vi "Memory Benchmark.vi"(5 "Show Cache Lines (F)":bool, 7 "Show Peak Bandwidth (F)":bool, 9 "Transfers (500)":i32=500, 10 "End Size":u64=50000000 format="%.0pB", 11 "Start Size":u64=1000 format="%.0pB") -> (3 "Memory Bandwidth":cluster{"X":dbl[], "Y":dbl[]}[](graph) caption="Memory Bandwidth Plot")   [LabVIEW 2017]
uses:
  Source/Classes/Pointer/Public/New/New (1B).vi
  Source/Classes/Pointer/Pointer.lvclass
panel:
  out "Peak Throughput":dbl format="%.3pB/s"
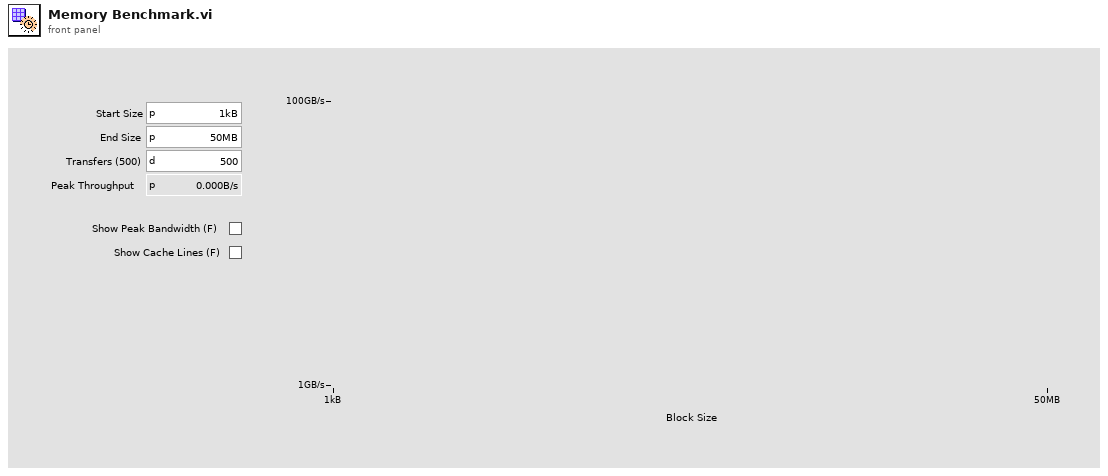
[diagram p1: front panel]
types:
  T1 = typedef "LVAnnotationListTypeDef.ctl" = cluster{"Name":string, "Color":u32, "Style":u8, "Point Style":u8, "Name Visible":bool, "Allow Drag":bool, "Annotation Mode":u32, "Plot":i32, "Index":i32, "Position":cluster{"X":dbl, "Y":dbl}, "X Scale":u32, "Y Scale":u32, "Show Arrow":bool, "Lock Name":bool, "Plot Area":i32, "Label Offset":cluster{"X":dbl, "Y":dbl}}[]
  T2 = cluster{"Name":string, "Color":u32, "Style":u8, "Point Style":u8, "Name Visible":bool, "Allow Drag":bool, "Annotation Mode":u32, "Plot":i32, "Index":i32, "Position":cluster{"X":dbl, "Y":dbl}, "X Scale":u32, "Y Scale":u32, "Show Arrow":bool, "Lock Name":bool, "Plot Area":i32, "Label Offset":cluster{"X":dbl, "Y":dbl}}
  T3 = cluster{"Name":string, "Color":u32, "Style":u8, "Point Style":u8, "Name Visible":bool, "Allow Drag":bool, "Annotation Mode":u32, "Plot":i32, "Index":i32, "Position":cluster{"X":dbl, "Y":dbl}, "X Scale":u32, "Y Scale":u32, "Show Arrow":bool, "Lock Name":bool, "Plot Area":i32, "Label Offset":cluster{"X":dbl, "Y":dbl}}[]
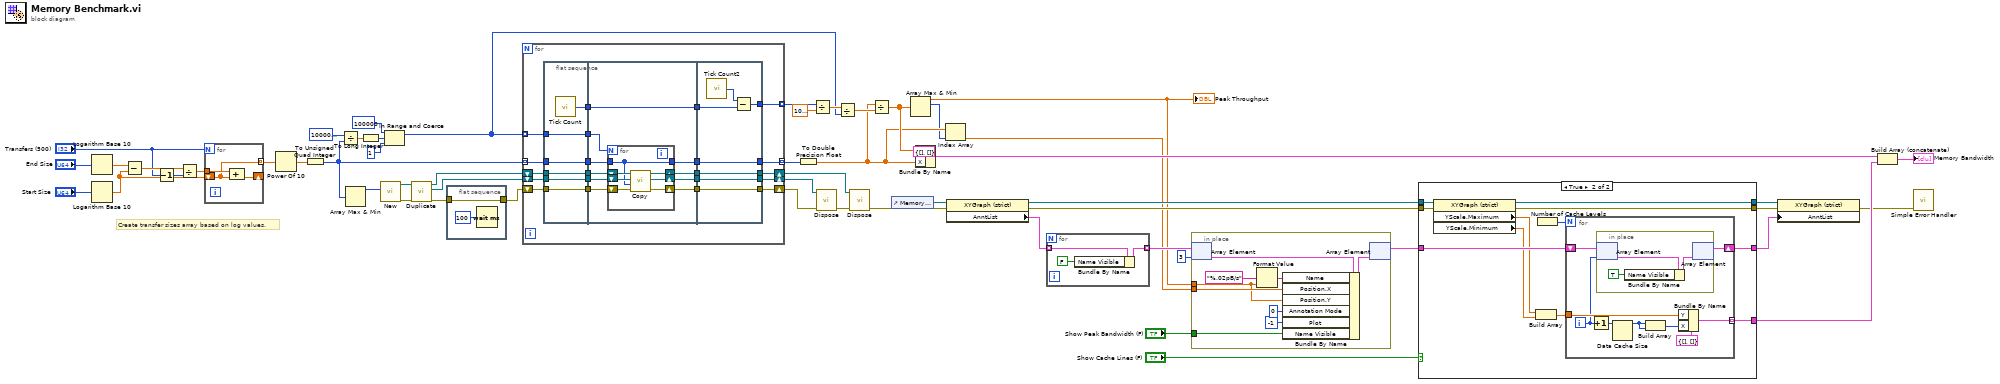
[diagram p0: block diagram]
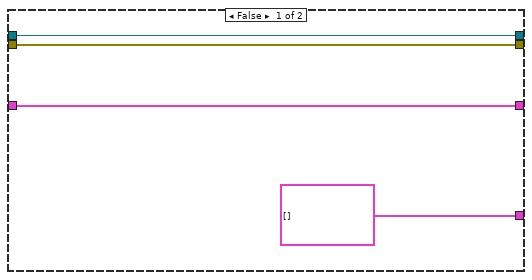
[diagram p2: hidden frame]
diagram:
  # "Create transfer sizes array based on log values."
  n1 = Logarithm Base 10(1:"End Size") -> (0:w54:dbl)
  n2 = Logarithm Base 10(1:"Start Size") -> (0:w51:dbl)
  n3 = Subtract(x=w54, y=w51) -> (x-y=w53:dbl)
  n4 = Decrement(x="Transfers (500)") -> (x-1=w49:i32)
  n5 = Divide(x=w53, y=w49) -> (x/y=w52:dbl)
  n6 = for {
    N: "Transfers (500)" -> [_]
    tunnel: w52 -> [w59]
    shift-right: [w58] -> _
    shift-left: w51 -> [w57]
    tunnel: [w57] -> w48 mode=indexing
    n7 = Compound Arithmetic op=ADD(w59, w57) -> (w58:dbl)
  }
  n8 = Power Of 10(x=w48) -> (10^x=w47:dbl[])
  n9 = To Unsigned Quad Integer(1:w47) -> (0:w41:u64[])
  n10 = Divide(x=u64 100000000, y=w41) -> (x/y=w40:dbl[])
  n11 = Array Max & Min(array=w41) -> (max value=w6:u64)  [unwired: 3 out]
  n12 = To Long Integer(number=w40) -> (32bit integer=w39:i32[])
  n13 = call-poly "New.vi"("count (1)"=w6) -> ("error out"=w36:errorcluster, "Pointer"=w3:refnum<class "Pointer.lvclass">)  [unwired: 9 in]
  n14 = In Range and Coerce(upper limit=100000, x=w39, lower limit=1) -> (coerced(x)=w20:i32[])  [unwired: 1 out]
  n15 = call "Duplicate.vi"("error in (no error)"=w36, "Pointer in"=w3) -> ("error out"=w26:errorcluster, "new duplicate Pointer"=w2:refnum<class "Pointer.lvclass">, "Pointer out"=w1:refnum<class "Pointer.lvclass">)  [unwired: 7 in]
  n16 = flat-sequence {
    tunnel: w26 -> [w61]
    tunnel: [w61] -> w25
    frame #0 {
      n17 = Wait (ms)(milliseconds to wait=u32 100) -> ()  [unwired: 1 out]
    }
  }
  n18 = for {
    shift-right: [w66] -> w34
    shift-left: w2 -> [w70]
    shift-right: [w65] -> w32
    shift-left: w1 -> [w69]
    shift-right: [w67] -> w35
    shift-left: w25 -> [w68]
    tunnel: [w64] -> w30 mode=indexing
    tunnel: w41 -> [w63] mode=indexing
    tunnel: [w62] -> w27 mode=indexing
    tunnel: w20 -> [w71] mode=indexing
    n19 = flat-sequence {
      tunnel: [w88] -> w82
      tunnel: [w87] -> w81
      tunnel: [w86] -> w80
      tunnel: [w85] -> w79
      tunnel: [w84] -> w78
      tunnel: [w83] -> w77
      tunnel: w69 -> [w88]
      tunnel: w70 -> [w87]
      tunnel: w68 -> [w86]
      tunnel: w63 -> [w85]
      tunnel: w71 -> [w84]
      tunnel: w82 -> [w98]
      tunnel: w81 -> [w89]
      tunnel: w80 -> [w97]
      tunnel: w79 -> [w96]
      tunnel: w78 -> [w92]
      tunnel: w77 -> [w91]
      tunnel: [w91] -> w76
      tunnel: [w95] -> w75
      tunnel: [w94] -> w74
      tunnel: [w93] -> w73
      tunnel: [w90] -> w72
      tunnel: w76 -> [w111]
      tunnel: w75 -> [w110]
      tunnel: w74 -> [w109]
      tunnel: w73 -> [w108]
      tunnel: w72 -> [w107]
      tunnel: [w110] -> w67
      tunnel: [w109] -> w65
      tunnel: [w108] -> w66
      tunnel: [w107] -> w62
      tunnel: [w106] -> w64
      frame #0 {
        n20 = call "Tick Count"() -> ("Tick Count(uSec)"=w83:u32)
      }
      frame #1 {
        n21 = for {
          N: w92 -> [_]
          shift-right: [w102] -> w95
          shift-left: w97 -> [w103]
          shift-right: [w101] -> w94
          shift-left: w98 -> [w105]
          shift-right: [w100] -> w93
          shift-left: w89 -> [w104]
          tunnel: w96 -> [w99]
          tunnel: [w99] -> w90
          n22 = call "Copy.vi"("error in (no error)"=w103, "bytes to copy"=w99, "dst Pointer in"=w104, "src Pointer in"=w105) -> ("error out"=w102:errorcluster, "dst Pointer out"=w100:refnum<class "Pointer.lvclass">, "src Pointer out"=w101:refnum<class "Pointer.lvclass">)  [unwired: 4 in, 1 out]
        }
      }
      frame #2 {
        n23 = call "Tick Count2"() -> ("Tick Count(uSec)"=w112:u32)
        n24 = Subtract(x=w112, y=w111) -> (x-y=w106:u32)
      }
    }
  }
  n25 = To Double Precision Float(number=w27) -> (double precision float=w24:dbl[])
  n26 = Divide(x=w30, y=1000000.0) -> (x/y=w29:dbl[])
  n27 = call "Dispose.vi"("error in (no error)"=w35, "Pointer in"=w34) -> ("error out"=w33:errorcluster)  [unwired: 8 in, 1 out]
  n28 = Divide(x=w29, y=w20) -> (x/y=w28:dbl[])
  n29 = call "Dispose.vi"("error in (no error)"=w33, "Pointer in"=w32) -> ("error out"=w10:errorcluster)  [unwired: 8 in, 1 out]
  n30 = Divide(x=w24, y=w28) -> (x/y=w46:dbl[])
  n31 = control-ref of="Memory Bandwidth"() -> (w18:refnum<vi>)
  n32 = Array Max & Min(array=w46) -> (max value=w12:dbl, max index (indices)=w22:i32)  [unwired: 2 out]
  "Peak Throughput" <- w12
  n33 = Bundle By Name(cluster=cluster{"X":dbl[], "Y":dbl[]} {"X"=[], "Y"=[]}, "Y"=w46, "X"=w24) -> (w44:cluster{"X":dbl[], "Y":dbl[]})
  n34 = Index Array(array=w24, index=w22) -> (element=w11:dbl)
  n35 = property class="XYGraph (strict)"(reference=w18, error in=w10) -> (reference out=w13:refnum<vi>, error out=w14:errorcluster, "AnntList"=w17:T1)
  n36 = for {
    tunnel: w17 -> [w114] mode=indexing
    tunnel: [w113] -> w15 mode=indexing
    n37 = Bundle By Name(cluster=w114, "Name Visible"=FALSE) -> (w113:T2)
  }
  n38 = in-place {
    in-place-border: w12 -> [w116]
    in-place-border: w11 -> [w120]
    in-place-border: "Show Peak Bandwidth (F)" -> [w117]
    n39 = in-place-array #1(w15, 3) -> (w124:T2)
    n40 = Format Value(format string="%.02pB/s", value (0)=w116) -> (output string=w122:string)  [unwired: 1 in]
    n41 = Bundle By Name(cluster=w124, "Name"=w122, "Position.X"=w120, "Position.Y"=w116, "Annotation Mode"=u32 0, "Plot"=-1, "Name Visible"=w117) -> (w121:T2)
    n42 = in-place-array #1(w121) -> (w19:T3)  [unwired: 1 out]
  }
  n43 = case shown="True" "Show Cache Lines (F)" {
    tunnel: [cluster{"X":dbl[], "Y":dbl[]}[] [] w137] -> w5
    tunnel: w13 -> [w125 w136]
    tunnel: w19 -> [w126 w135]
    tunnel: w14 -> [w127 w134]
    tunnel: [w127 w131] -> w9
    tunnel: [w125 w130] -> w8
    tunnel: [w126 w129] -> w7
    frame False {
    }
    frame True {
      n44 = property class="XYGraph (strict)"(reference=w136, error in=w134) -> (reference out=w130:refnum<vi>, error out=w131:errorcluster, "YScale.Maximum"=w133:dbl, "YScale.Minimum"=w132:dbl)
      n45 = Build Array(w133, w132) -> (w138:dbl[])
      n46 = Number of Cache Levels() -> (w139:i32)
      n47 = for {
        N: w139 -> [_]
        tunnel: w138 -> [w144]
        tunnel: [w143] -> w137 mode=indexing
        shift-right: [w141] -> w129
        shift-left: w135 -> [w142]
        i -> [w140]
        n48 = Increment(x=w140) -> (x+1=w148:i32)
        n49 = in-place {
          n50 = in-place-array #2(w142, w140) -> (w151:T2)
          n51 = Bundle By Name(cluster=w151, "Name Visible"=TRUE) -> (w150:T2)
          n52 = in-place-array #2(w150) -> (w141:T3)  [unwired: 1 out]
        }
        n53 = Data Cache Size(0:w148) -> (4:w146:i32)  [unwired: 1 out]
        n54 = Build Array(w146, w146) -> (w145:i32[])
        n55 = Bundle By Name(cluster=cluster{"X":dbl[], "Y":dbl[]} {"X"=[], "Y"=[]}, "Y"=w144, "X"=w145) -> (w143:cluster{"X":dbl[], "Y":dbl[]})
      }
    }
  }
  n56 = property class="XYGraph (strict)"(reference=w8, error in=w9, "AnntList"=w7) -> (error out=w4:errorcluster)  [unwired: 1 out]
  n57 = Build Array (concatenate)(w44, w5) -> (→"Memory Bandwidth":cluster{"X":dbl[], "Y":dbl[]}[])
  n58 = call <vilib>:"Simple Error Handler.vi"("error in (no error)"=w4) -> ()  [unwired: 4 in, 5 out]
